vi "Terminate.vi"(0 "Session Handle in":T1, 11 "error in (no error)":errorcluster) -> (4 "Session Handle out":T1, 15 "error out":errorcluster)   [LabVIEW 2019, in "HTS.lvlib" / "Execution.lvclass"]
uses:
  Execution.lvclass
  Typedefs/Session Handle.ctl
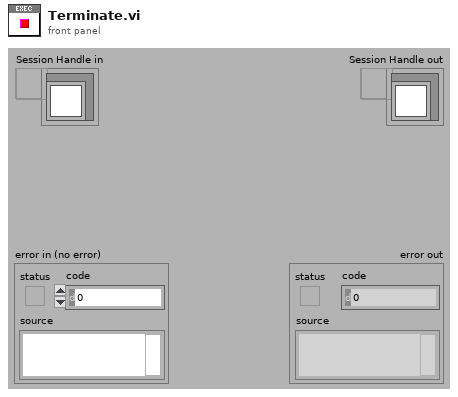
[diagram p1: front panel]
types:
  T1 = typedef "HTS.lvlib/Execution.lvclass/Session Handle.ctl" = refnum<data-value>
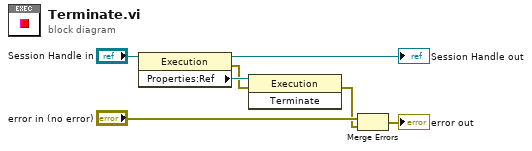
[diagram p0: block diagram]
diagram:
  n1 = property class="Execution"(reference="Session Handle in") -> (reference out=→"Session Handle out":T1, error out=w3:errorcluster, "Properties:Ref"=w4:refnum<k7>)  [unwired: 1 in]
  n2 = invoke class="Execution" method="Terminate"(reference=w4, error in=w3) -> (error out=w1:errorcluster)  [unwired: 1 in, 2 out]
  n3 = Merge Errors("error in (no error)", w1) -> (→"error out":errorcluster)
